vi "testClearErrorAndSendExplanation.vi"(8 "error in (no error)":errorcluster) -> (0 "error out":errorcluster)   [LabVIEW 2018]
doc: "Test the clearErrorAndSendExplanation.vi."
uses:
  src/TcpServerBase/typedef/msgTypeDef.ctl
  src/TcpServerBase/TcpServerBase.lvclass
  src/TcpServerBase/TcpServerBase.lvclass/TcpServerBase.ctl
  <vilib>/addons/_JKI Toolkits/Caraya/classes/Assert/Assert Not Equal Value_Variant.vi
  <vilib>/addons/_JKI Toolkits/Caraya/classes/Test/Test.lvclass
  <vilib>/addons/_JKI Toolkits/Caraya/classes/Assert/Assert.lvclass
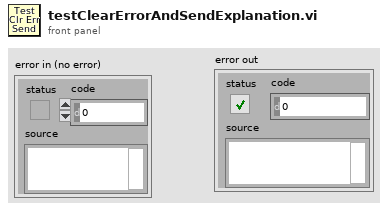
[diagram p1: front panel]
types:
  T1 = typedef "TcpServerBase.lvclass/msgTypeDef.ctl" = cluster{"msgName":string, "msgDetails":string}
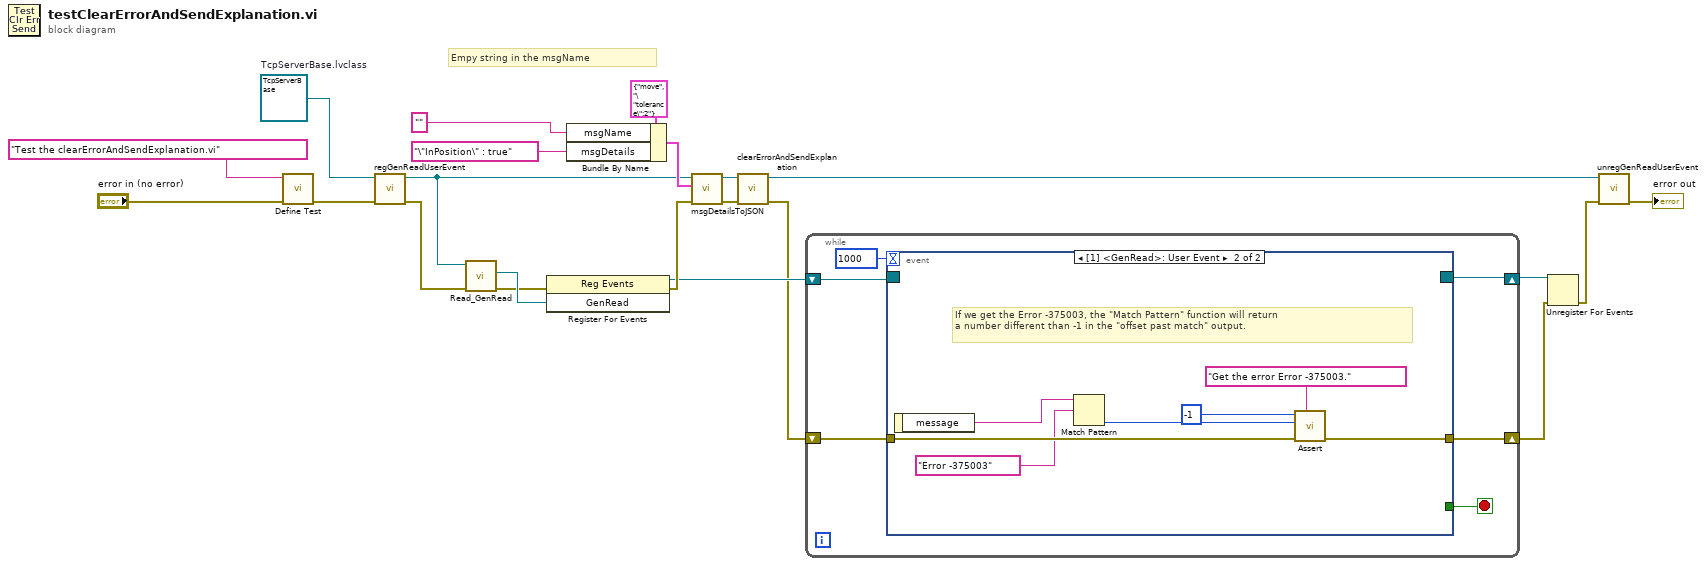
[diagram p0: block diagram]
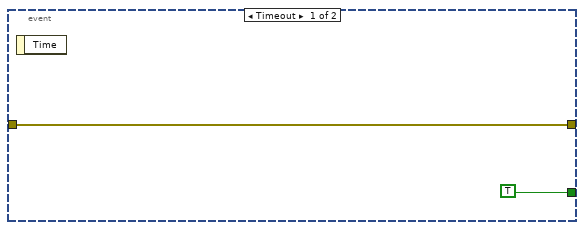
[diagram p2: hidden frame]
diagram:
  w16 = refnum<class "TcpServerBase.lvclass"> refnum  # TcpServerBase.lvclass
  # "Empy string in the msgName"
  n1 = call <vilib>:"Define Test.vi"("error in (no error)"="error in (no error)", "Label (VI Title)"="Test the clearErrorAndSendExplanation.vi") -> ("error out"=w15:errorcluster)  [unwired: 9 in]
  n2 = call "regGenReadUserEvent.vi"("error in (no error)"=w15, "TcpServerBase in"=w16) -> ("error out"=w14:errorcluster, "TcpServerBase out"=w4:refnum<class "TcpServerBase.lvclass">)  [unwired: 8 in]
  n3 = call "Read_GenRead.vi"("error in (no error)"=w14, "TcpServerBase in"=w4) -> ("error out"=w11:errorcluster, "GenRead"=w13:refnum<user-event>)  [unwired: 7 in, 1 out]
  n4 = register-events(error in=w11, w13) -> (reference out=w10:refnum<event-registration>, error out=w12:errorcluster)  [unwired: 1 in]
  n5 = Bundle By Name(cluster=T1 {"msgName"="move", "msgDetails"="\"tolerance\":2"} ("msgTypeDef"), "msgName"="" ("String"), "msgDetails"="\"InPosition\" : true" ("String")) -> (w19:T1)
  n6 = call "msgDetailsToJSON.vi"("error in (no error)"=w12, "msgData"=w19, "TcpServerBase in"=w4) -> ("error out"=w5:errorcluster, "TcpServerBase out"=w2:refnum<class "TcpServerBase.lvclass">)  [unwired: 6 in, 1 out]
  n7 = call "clearErrorAndSendExplanation.vi"("error in (no error)"=w5, "TcpServerBase in"=w2) -> ("error out"=w3:errorcluster, "TcpServerBase out"=w1:refnum<class "TcpServerBase.lvclass">)  [unwired: 8 in]
  n8 = while {
    shift-right: [w25] -> w8
    shift-left: w3 -> [w23]
    shift-right: [w24] -> w9
    shift-left: w10 -> [w26]
    stop <- w27 stop-if-true
    n9 = event shown="[1] <GenRead>: User Event" {
      selector: w26 -> [_ _]
      dyn-events: [_ _] -> w24
      timeout: 1000 -> [_ _]
      tunnel: [TRUE _] -> w27
      tunnel: [w29 w36] -> w25
      tunnel: w23 -> [w29 w35]
      event Timeout {
        n10 = event-data() -> ()  [unwired: 1 in, 1 out]
      }
      event User Event {
        # "If we get the Error -375003, the \"Match Pattern\" function will return\na number different than -1 in the \"offset past match\" output."
        n11 = event-data() -> ("message"=w34:string)  [unwired: 1 in]
        n12 = Match Pattern(string=w34, regular expression="Error -375003" ("error string")) -> (offset past match=w31:i32)  [unwired: 1 in, 3 out]
        n13 = call-poly <vilib>:"Assert.vi"("Label"="Get the error Error -375003.", "error in (no error)"=w35, "Y"=w31, "X"=-1 ("offset past match")) -> ("error out"=w36:errorcluster)  [unwired: 7 in]
      }
    }
  }
  n14 = Unregister For Events(event registration refnum=w9, error in=w8) -> (error out=w7:errorcluster)
  n15 = call "unregGenReadUserEvent.vi"("error in (no error)"=w7, "tcpServerBase in"=w1) -> ("error out"=→"error out":errorcluster)  [unwired: 8 in, 1 out]
